vi "Run 2 Stimuli.vi"() -> ()   [LabVIEW 2015]
uses:
  Ramp Stimulus/Ramp Stimulus.lvclass
  Sine Stimulus/Sine Stimulus.lvclass
  Stimulus/Stimulus.lvclass
panel:
  out "Waveform Graph":dbl[][](graph)
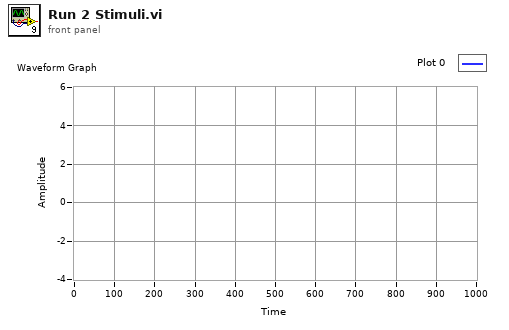
[diagram p1: front panel]
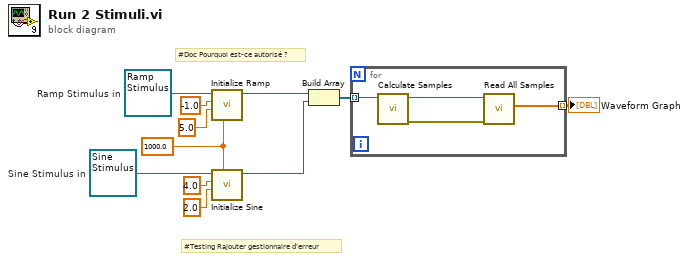
[diagram p0: block diagram]
diagram:
  w3 = 1000.0 ("Sample Count")
  w6 = refnum<class "Sine Stimulus.lvclass"> refnum  # Sine Stimulus in
  w7 = refnum<class "Ramp Stimulus.lvclass"> refnum  # Ramp Stimulus in
  # "#Doc Pourquoi est-ce autorisé ?"
  # "#Testing Rajouter gestionnaire d'erreur"
  n1 = call-dynamic "Initialize Ramp.vi"("Sample Count"=w3, "End"=5.0, "Start"=-1.0, "Ramp Stimulus in"=w7) -> ("Ramp Stimulus out"=w11:refnum<class "Ramp Stimulus.lvclass">)  [unwired: 6 in, 1 out]
  n2 = call-dynamic "Initialize Sine.vi"("Sample Count"=w3, "Frequency"=2.0, "Amplitude"=4.0, "Sine Stimulus in"=w6) -> ("Sine Stimulus out"=w10:refnum<class "Sine Stimulus.lvclass">)  [unwired: 6 in, 1 out]
  n3 = Build Array(w11, w10) -> (w9:refnum<class "Stimulus.lvclass">[])
  n4 = for {
    tunnel: w9 -> [w14] mode=indexing
    tunnel: [w15] -> w8 mode=indexing
    n5 = call-dynamic "Calculate Samples.vi"("Stimulus in"=w14) -> ("error out"=w12:errorcluster, "Stimulus out"=w13:refnum<class "Stimulus.lvclass">)  [unwired: 9 in]
    n6 = call-dynamic "Read All Samples.vi"("error in (no error)"=w12, "Stimulus in"=w13) -> ("All Samples"=w15:dbl[])  [unwired: 7 in, 2 out]
  }
  "Waveform Graph" <- w8
